vi "LimeLight targeting.vi"(8 "error in (no error)":errorcluster) -> (0 "error out":errorcluster)   [LabVIEW 2023]
uses:
  ctrl defs/ctrl LimeLight target.ctl
  Global odometry.vi
  <vilib>/Rock Robotics/Network Tables/NT Read Number.vi
panel:
  in  "Limelight target\ntest input":T1={"offsetAngle H"=10.0, "offsetAngle V"=27.0, "area"=0.0, "skew"=0.0, "driver assist"=FALSE}
  in  "testing?":bool
  out "distance":dbl=16.17019952446243
  out "d from dV":dbl=15.92453785944492
  in  "target ht (in)":dbl=48.0
  in  "cameraAngle (deg)":dbl=10.0
  in  "camera ht (in)":dbl=36.0
  out "LimeLight\ntargeting data":T1={"offsetAngle H"=10.0, "offsetAngle V"=27.0, "area"=0.0, "skew"=0.0, "driver assist"=FALSE}
  in  "stop":bool
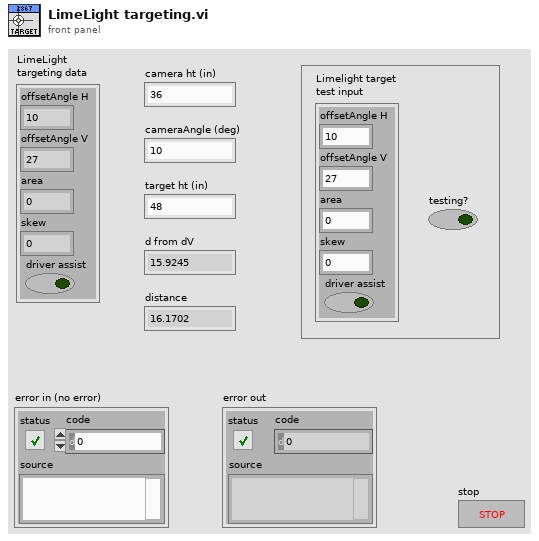
[diagram p1: front panel]
types:
  T1 = typedef "ctrl LimeLight target.ctl" = cluster{"offsetAngle H":dbl, "offsetAngle V":dbl, "area":dbl, "skew":dbl, "driver assist":bool}
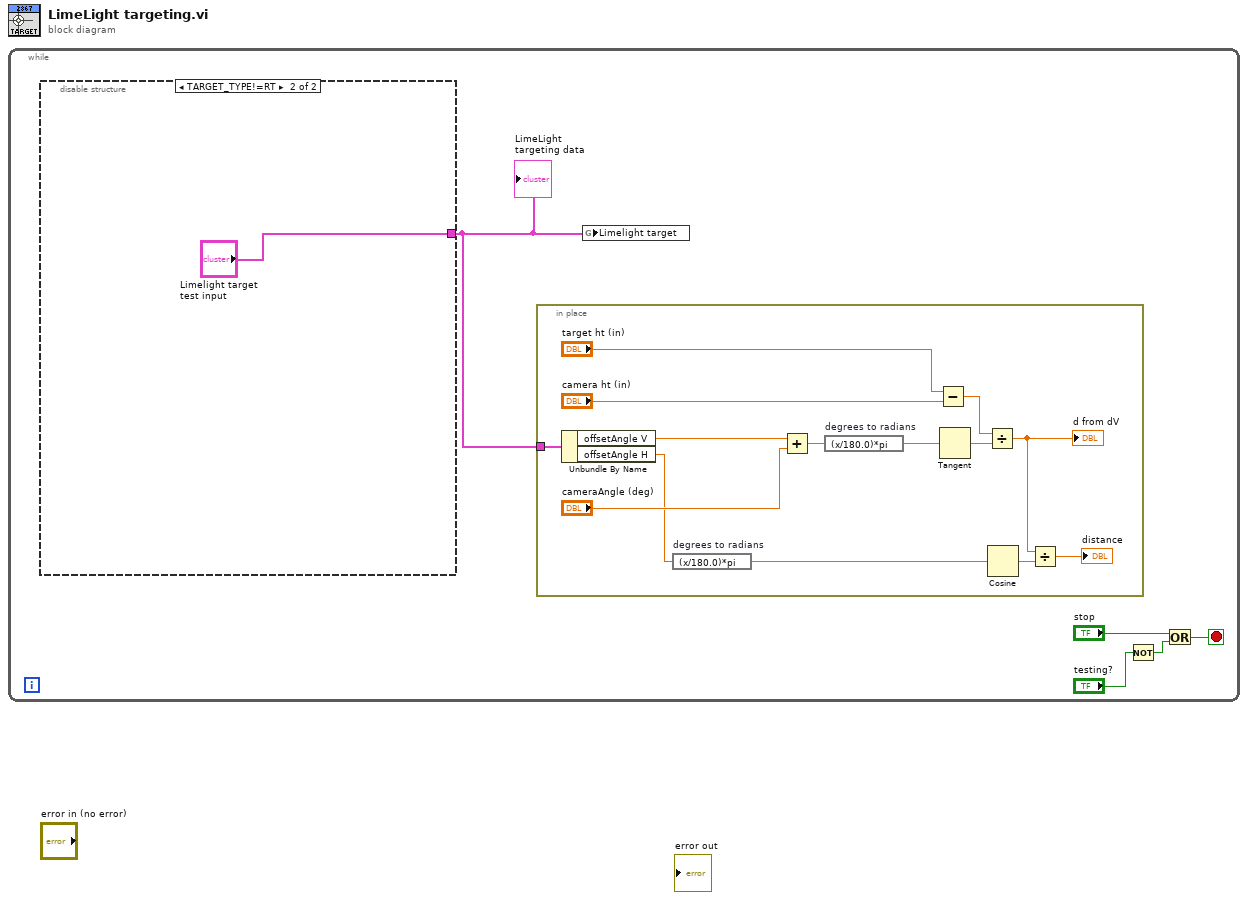
[diagram p0: block diagram]
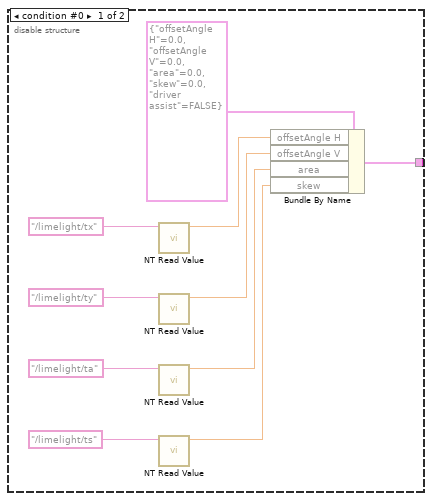
[diagram p2: hidden frame]
diagram:
  n1 = while {
    stop <- w2 stop-if-true
    n2 = disable-structure shown="TARGET_TYPE!=RT" {
      disable-tunnel: [w20 "Limelight target\ntest input"] -> w3
      frame condition #0 {
        n3 = call-poly <vilib>:"NT Read Value.vi"("name"="/limelight/tx") -> ("value"=w24:dbl)  [unwired: 8 in, 2 out]
        n4 = call-poly <vilib>:"NT Read Value.vi"("name"="/limelight/ty") -> ("value"=w23:dbl)  [unwired: 8 in, 2 out]
        n5 = call-poly <vilib>:"NT Read Value.vi"("name"="/limelight/ta") -> ("value"=w22:dbl)  [unwired: 8 in, 2 out]
        n6 = call-poly <vilib>:"NT Read Value.vi"("name"="/limelight/ts") -> ("value"=w21:dbl)  [unwired: 8 in, 2 out]
        n7 = Bundle By Name(cluster=T1 {"offsetAngle H"=0.0, "offsetAngle V"=0.0, "area"=0.0, "skew"=0.0, "driver assist"=FALSE} ("Limelight target"), "offsetAngle H"=w24, "offsetAngle V"=w23, "area"=w22, "skew"=w21) -> (w20:T1)
      }
      frame condition #1 (active) {
      }
    }
    "LimeLight\ntargeting data" <- w3
    n8 = in-place {
      in-place-border: w3 -> [w16]
      n9 = Unbundle By Name(w16) -> ("offsetAngle V"=w15:dbl, "offsetAngle H"=w9:dbl)
      n10 = expression code="(x/180.0)*pi" "degrees to radians"(w9) -> (w10:dbl)
      n11 = Add(x=w15, y="cameraAngle (deg)") -> (x+y=w13:dbl)
      n12 = expression code="(x/180.0)*pi" "degrees to radians"(w13) -> (w12:dbl)
      n13 = Subtract(x="target ht (in)", y="camera ht (in)") -> (x-y=w17:dbl)
      n14 = Tangent(1:w12) -> (0:w11:dbl)
      n15 = Divide(x=w17, y=w11) -> (x/y=w8:dbl)
      "d from dV" <- w8
      n16 = Cosine(x=w10) -> (cos(x)=w7:dbl)
      n17 = Divide(x=w8, y=w7) -> (x/y=→"distance":dbl)
    }
    n18 = global write "Global odometry.vi" "Limelight target"(w3) -> ()
    n19 = Not(x="testing?") -> (.not. x?=w5:bool)
    n20 = Or(x="stop", y=w5) -> (x .or. y?=w2:bool)
  }
